vi "Pre Launch Init.vi"(11 "SubPanel Actor in":refnum<class "SubPanel Actor.lvclass">) -> (0 "error out":errorcluster, 3 "SubPanel Actor out":refnum<class "SubPanel Actor.lvclass">)   [LabVIEW 2020, in "SubPanel Actor.lvlib" / "SubPanel Actor.lvclass"]
doc: "(<B>Filename</B>: Actor Framework.lvlib:Actor.lvclass:Pre Launch Init.vi)\n\nDefines behavior that occurs after the Launch Nested Actor method is invoked but before the actor's Actor Core method begins running.\n\nBy default, this method does nothing. A descendant class may override it to define behavior."
uses:
  SubPanel Actor.lvclass
  C:/Program Files (x86)/National Instruments/LabVIEW 2020/vi.lib/ActorFramework/Actor/Actor.lvclass
  <vilib>/ActorFramework/Actor/Actor.lvclass/Actor.ctl
  <vilib>/ActorFramework/Message Enqueuer/Message Enqueuer.lvclass/Message Enqueuer.ctl
  <vilib>/ActorFramework/Message Enqueuer/Init from Existing Queue.vi
  <vilib>/ActorFramework/Message Enqueuer/Enqueue.vi
  SubPanel Actor Messages/Initialize Msg/Initialize Msg.lvclass
  C:/Program Files (x86)/National Instruments/LabVIEW 2020/vi.lib/ActorFramework/Message/Message.lvclass
  <vilib>/ActorFramework/Message Priority Queue/Priority Enqueue.vi
  <vilib>/ActorFramework/Actor/Actor.lvclass
  <vilib>/ActorFramework/Message Enqueuer/Message Enqueuer.lvclass
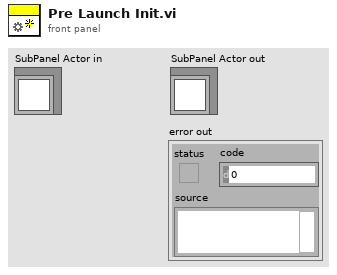
[diagram p1: front panel]
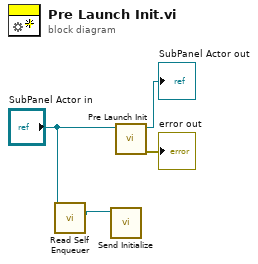
[diagram p0: block diagram]
diagram:
  n1 = call <vilib>:"Read Self Enqueuer.vi"("Actor"="SubPanel Actor in") -> ("Self Enqueuer"=w2:refnum<class "Message Enqueuer.lvclass">)  [unwired: 10 in]
  n2 = call "Send Initialize.vi"("Message Enqueuer"=w2) -> ()  [unwired: 9 in, 2 out]
  n3 = call-parent "Pre Launch Init.vi"("Actor in"="SubPanel Actor in") -> ("error out"=→"error out":errorcluster, "Actor out"=→"SubPanel Actor out":refnum<class "SubPanel Actor.lvclass">)  [unwired: 9 in]
